vi "Inficon - Set final thickness.vi"(8 "Error In":errorcluster, 10 "Final Thickness":dbl min=0.0 max=999.0 step=0.001 format="%.;%.3f", 11 "COM in":refnum<visa-resource-name>) -> (0 "Error Out":errorcluster, 3 "COM out":refnum<visa-resource-name>)   [LabVIEW 2016]
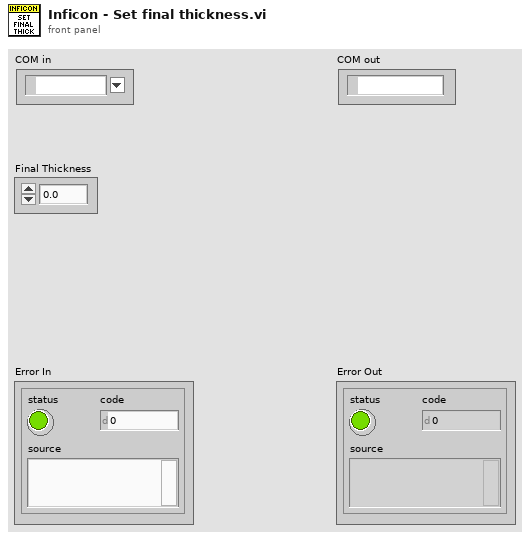
[diagram p1: front panel]
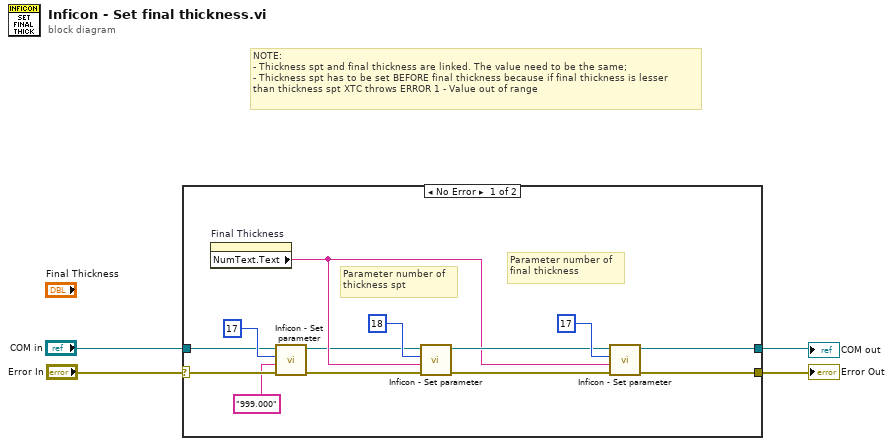
[diagram p0: block diagram]
diagram:
  # "NOTE: \n- Thickness spt and final thickness are linked. The value need to be the same;\n- Thickness spt has to be set BEFORE final thickness because if final thickness is lesser\nthan thickness spt XTC throws ERROR 1 - Value out of range"
  n1 = case shown="No Error" "Error In" {
    selector: "Error In" -> [w8 w18]
    tunnel: [w17 w18] -> w3
    tunnel: "COM in" -> [w9 w19]
    tunnel: [w16 w19] -> w1
    frame No Error {
      # "Parameter number of\nthickness spt"
      # "Parameter number of\nfinal thickness"
      n2 = property on="Final Thickness" class="DigNum (strict)"() -> ("NumText.Text"=w11:string)  [unwired: 2 in, 2 out]
      n3 = call "Inficon - Set parameter.vi"("Error In"=w8, "Param value"="999.000", "Param number"=u8 17, "COM in"=w9) -> ("Error Out"=w7:errorcluster, "COM out"=w6:refnum<visa-resource-name>)  [unwired: 6 in]
      n4 = call "Inficon - Set parameter.vi"("Error In"=w7, "Param value"=w11, "Param number"=u8 18, "COM in"=w6) -> ("Error Out"=w12:errorcluster, "COM out"=w13:refnum<visa-resource-name>)  [unwired: 6 in]
      n5 = call "Inficon - Set parameter.vi"("Error In"=w12, "Param value"=w11, "Param number"=u8 17, "COM in"=w13) -> ("Error Out"=w17:errorcluster, "COM out"=w16:refnum<visa-resource-name>)  [unwired: 6 in]
    }
    frame Error {
    }
  }
  "Error Out" <- w3
  "COM out" <- w1
